vi "main.vi"() -> ()   [LabVIEW 2015]
uses:
  <vilib>/Utility/inputDevices.llb/keyboardAcquire.vi
  <vilib>/Utility/inputDevices.llb/closeKeyboard.vi
panel:
  out "PIANO":bool[](array[boolean])
  out "keys pressed":T1(array[ring])
  out "CONFIG":string[](array[string])
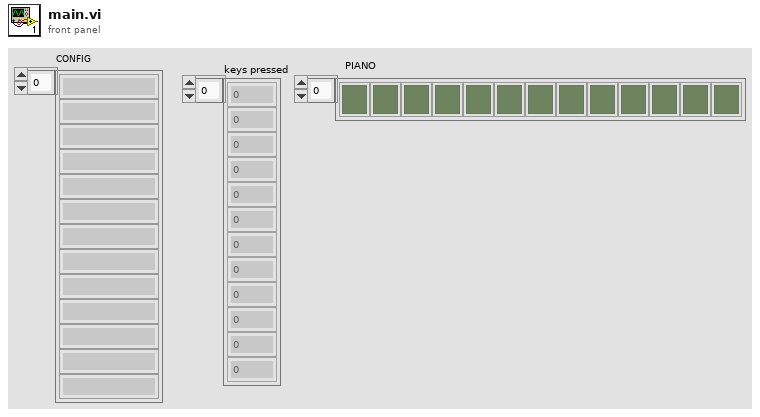
[diagram p1: front panel]
types:
  T1 = enum16{"0", "1", "2", "3", "4", "5", "6", "7", "8", "9", "A", "B", "C", "D", "E", "F", "G", "H", "I", "J", "K", "L", "M", "N", "O", "P", "Q", "R", "S", "T", "U", "V", "W", "X", "Y", "Z", "F1", "F2", "F3", "F4", "F5", "F6", "F7", "F8", "F9", "F10", "F11", "F12", "F13", "F14", "F15", "ADD", "BACK", "BACKSLASH", "CAPITAL", "COMMA", "DECIMAL", "DELETE", "DIVIDE", "DOWN", "END", "EQUALS", "ESCAPE", "GRAVE (`)", "HOME", "INSERT", "LBRACKET", "LCONTROL", "LEFT", "L ALT", "LSHIFT", "LWIN", "MINUS", "MULTIPLY", "NEXT", "NUMLOCK", "NUMPAD_0", "NUMPAD_1", "NUMPAD_2", "NUMPAD_3", "NUMPAD_4", "NUMPAD_5", "NUMPAD_6", "NUMPAD_7", "NUMPAD_8", "NUMPAD_9", "PAUSE", "PERIOD", "PRIOR (PG UP)", "RBRACKET", "RCONTROL", "RETURN", "RIGHT", "R ALT", "RSHIFT", "RWIN", "SCROLL", "SEMICOLON", "SLASH", "SPACE", "SUBTRACT", "TAB", "UP", "ENTER (num pad)", "' (quote)"}[]
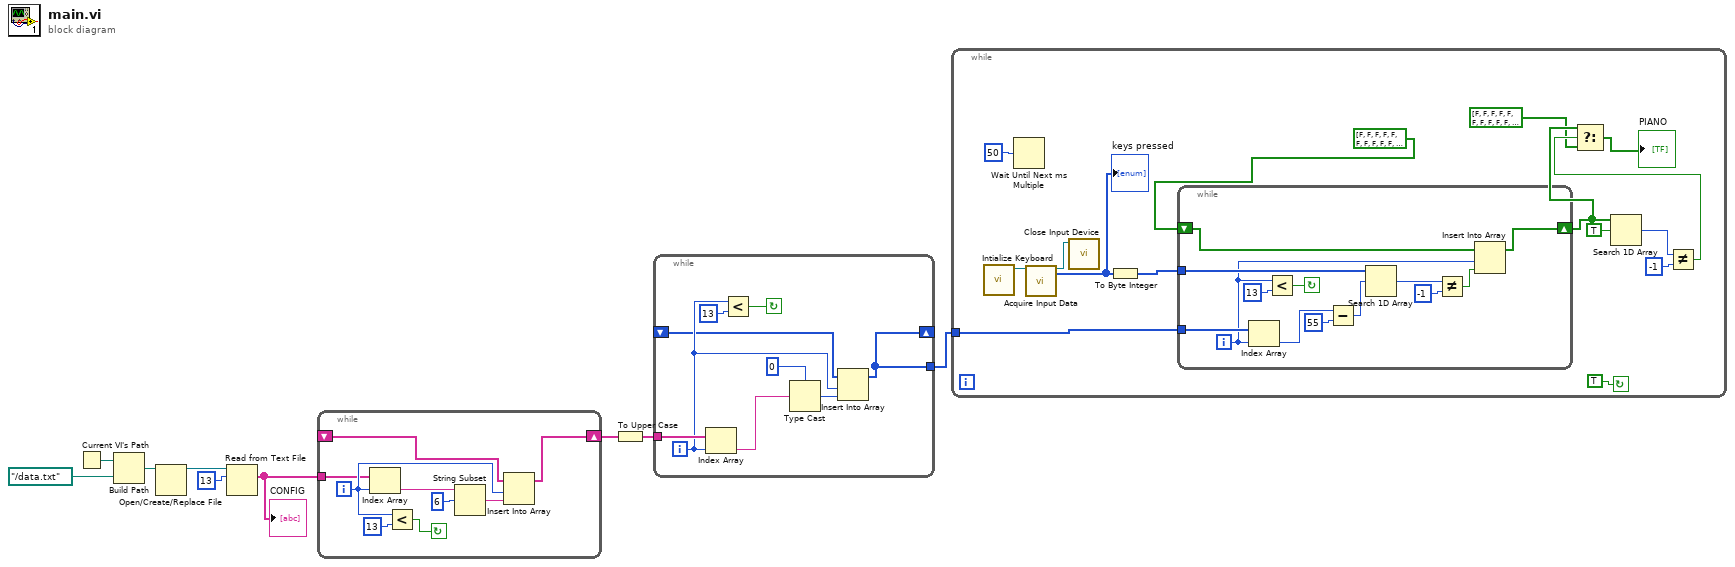
[diagram p0: block diagram]
diagram:
  n1 = Current VI's Path() -> (path=w6:path)
  n2 = Build Path(base path=w6, name or relative path=path "../data.txt") -> (appended path=w7:path)
  n3 = Open/Create/Replace File(file path (use dialog)=w7) -> (refnum out=w9:refnum<file>)  [unwired: 5 in, 2 out]
  n4 = Read from Text File(file (use dialog)=w9, count=13) -> (text=w4:string[])  [unwired: 2 in, 3 out]
  "CONFIG" <- w4
  n5 = while {
    tunnel: w4 -> [w12]
    shift-right: [w10] -> w3
    shift-left: _ -> [w11]
    i -> [w16]
    stop <- w17 continue-if-true
    n6 = Index Array(array=w12, index=w16) -> (element=w15:string)
    n7 = Less?(x=w16, y=13) -> (x < y?=w17:bool)
    n8 = String Subset(string=w15, offset (0)=6) -> (substring=w13:string)  [unwired: 1 in]
    n9 = Insert Into Array(array=w11, index=w16, new element=w13) -> (w10:string[])
  }
  n10 = To Upper Case(1:w3) -> (0:w2:string[])
  n11 = while {
    tunnel: w2 -> [w25]
    shift-right: [w19] -> _
    shift-left: _ -> [w20]
    tunnel: [w19] -> w1
    i -> [w22]
    stop <- w26 continue-if-true
    n12 = Index Array(array=w25, index=w22) -> (element=w24:string)
    n13 = Less?(x=w22, y=13) -> (x < y?=w26:bool)
    n14 = Type Cast(type=i8 0, x=w24) -> (*(type *) &x=w21:i8)
    n15 = Insert Into Array(array=w20, index=w22, new element=w21) -> (w19:i8[])
  }
  n16 = while {
    tunnel: w1 -> [w37]
    stop <- TRUE continue-if-true
    n17 = call <vilib>:"Intialize Keyboard.vi"() -> ("device ID"=w42:refnum<k1>)  [unwired: 10 in, 1 out]
    n18 = Wait Until Next ms Multiple(millisecond multiple=u32 50) -> ()  [unwired: 1 out]
    n19 = call-poly <vilib>:"Acquire Input Data.vi"("device ID"=w42) -> ("device ID"=w41:refnum<k1>, "keys pressed"=w38:T1)  [unwired: 16 in, 1 out]
    "keys pressed" <- w38
    n20 = call-poly <vilib>:"Close Input Device.vi"("device ID"=w41) -> ()  [unwired: 9 in, 1 out]
    n21 = To Byte Integer(number=w38) -> (8bit integer=w36:i8[])
    n22 = while {
      tunnel: w36 -> [w51]
      tunnel: w37 -> [w53]
      shift-right: [w44] -> w31
      shift-left: bool[] [FALSE, FALSE, FALSE, FALSE, FALSE, FALSE, FALSE, FALSE, FALSE, FALSE, FALSE, FALSE, FALSE] ("f") -> [w43]
      i -> [w47]
      stop <- w54 continue-if-true
      n23 = Index Array(array=w53, index=w47) -> (element=w52:i8)
      n24 = Less?(x=w47, y=13) -> (x < y?=w54:bool)
      n25 = Subtract(x=w52, y=i8 55) -> (x-y=w50:i8)
      n26 = Search 1D Array(1D array=w51, element=w50) -> (index of element=w46:i32)  [unwired: 1 in]
      n27 = Not Equal?(x=w46, y=-1) -> (x != y?=w45:bool)
      n28 = Insert Into Array(array=w43, index=w47, new element=w45) -> (w44:bool[])
    }
    n29 = Search 1D Array(1D array=w31, element=TRUE) -> (index of element=w33:i32)  [unwired: 1 in]
    n30 = Not Equal?(x=w33, y=-1) -> (x != y?=w32:bool)
    n31 = Select(t=w31, s=w32, f=bool[] [FALSE, FALSE, FALSE, FALSE, FALSE, FALSE, FALSE, FALSE, FALSE, FALSE, FALSE, FALSE, TRUE]) -> (s? t:f=→"PIANO":bool[])
  }
